vi "DQMH_Get Module ID.vi"(10 "Modules":T1, 11 "Module Name":string) -> (3 "Module ID out":i32)   [LabVIEW 2025]
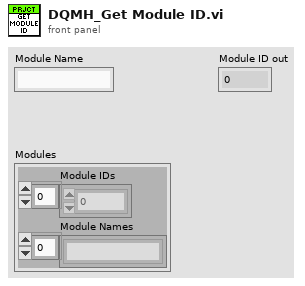
[diagram p1: front panel]
types:
  T1 = cluster{"Module IDs":i32[], "Module Names":string[]}
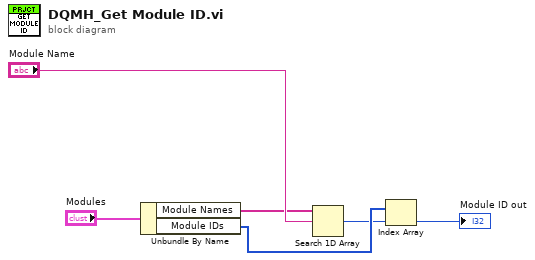
[diagram p0: block diagram]
diagram:
  n1 = Unbundle By Name("Modules") -> ("Module Names"=w2:string[], "Module IDs"=w5:i32[])
  n2 = Search 1D Array(1D array=w2, element="Module Name") -> (index of element=w4:i32)  [unwired: 1 in]
  n3 = Index Array(array=w5, index=w4) -> (element=→"Module ID out":i32)
